vi "Actor Core.vi"(8 "error in":errorcluster, 11 "Select Report File Dialog in":refnum<class "Display Settings Dialog.lvclass">) -> (0 "error out":errorcluster, 3 "Actor out":refnum<class "Actor.lvclass">)   [LabVIEW 2014, in "Display Settings Dialog.lvlib" / "Display Settings Dialog.lvclass"]
doc: "(<B>Filename</B>: Actor Framework.lvlib:Actor.lvclass:Actor Core.vi)\n\nReceives messages to the actor, reacts to them, and initiates any error handling that may shut the actor down.\n\nDescendant classes may override this VI to append parallel tasks for the actor to complete while it handles messages. Overrides use the Call Parent Method node."
uses:
  Display Settings Dialog.lvclass
  <vilib>/ActorFramework/Actor/Actor.lvclass
  HIJ Vision Display/HIJ Vision Display/DisplaySettings.ctl
  <vilib>/ActorFramework/Actor/Actor.lvclass/Actor.ctl
  <vilib>/ActorFramework/Message Enqueuer/Message Enqueuer.lvclass/Message Enqueuer.ctl
  Display Settings Dialog.lvclass/Display Settings Dialog.ctl
  Display Settings Dialog Messages/Write Display settings Msg/Write Display settings Msg.lvclass/Write Display settings Msg.ctl
  HIJ Vision Display/HIJ Vision Display Messages/New Dispay Settings Msg/New Dispay Settings Msg.lvclass/New Dispay Settings Msg.ctl
  <vilib>/ActorFramework/Message Enqueuer/Init from Existing Queue.vi
  <vilib>/ActorFramework/Message Enqueuer/Enqueue.vi
  <vilib>/ActorFramework/Message Priority Queue/Priority Enqueue.vi
  <vilib>/ActorFramework/Message Enqueuer/Message Enqueuer.lvclass
  Display Settings Dialog Messages/Write Display settings Msg/Write Display settings Msg.lvclass
  HIJ Vision Display/HIJ Vision Display Messages/New Dispay Settings Msg/New Dispay Settings Msg.lvclass
  <vilib>/ActorFramework/Stop Msg/Stop Msg.lvclass
  Shared Code/Viewable Actor/ViewableActor/ViewableActor.lvclass
  HIJ Vision Display/HIJ Vision Display/HIJ Vision Display.lvclass
panel:
  in  "Display settings":T1={"Min. Thresh."=0.0, "X"=0.0, "Y"=0.0, "ShowLineout"=FALSE, "ScaleParts"=10, "ShowLegende"=FALSE, "Target Cross"=FALSE, "Centroid Cross"=FALSE, "Target color"=16777226, "Centroid color"=16711680, "calibr. µm/px"=0.0}
  in  "Stop Signal":bool
  in  "Stop":bool
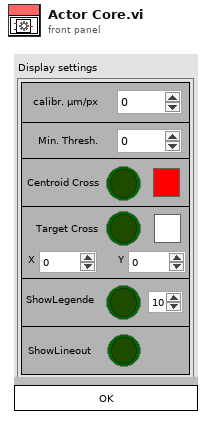
[diagram p1: front panel]
types:
  T1 = typedef "HIJ Vision Display.lvlib/HIJ Vision Display.lvclass/DisplaySettings.ctl" = cluster{"Min. Thresh.":sgl, "X":dbl, "Y":dbl, "ShowLineout":bool, "ScaleParts":i32, "ShowLegende":bool, "Target Cross":bool, "Centroid Cross":bool, "Target color":u32, "Centroid color":u32, "calibr. µm/px":sgl[unit]}
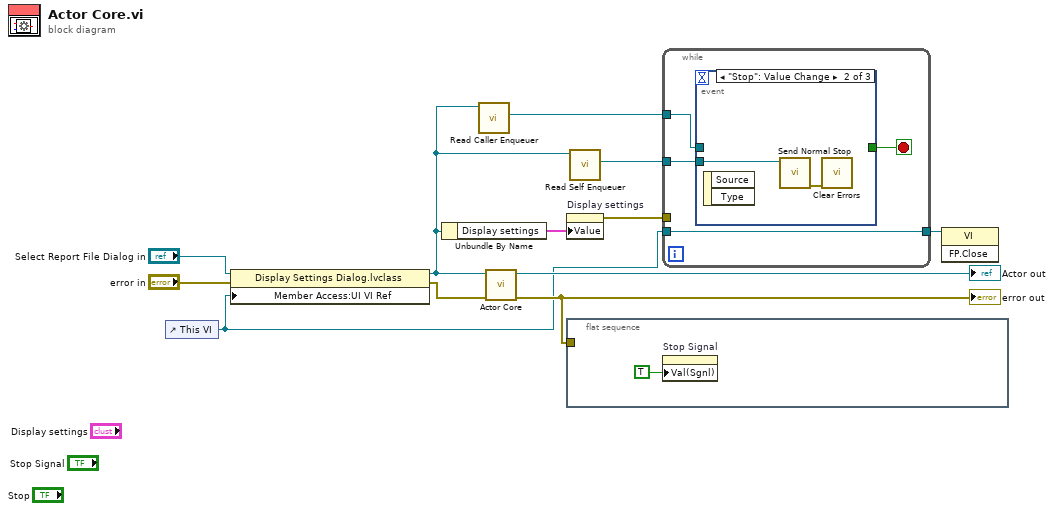
[diagram p0: block diagram]
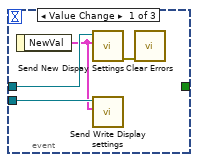
[diagram p2: hidden frame]
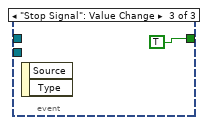
[diagram p3: hidden frame]
diagram:
  n1 = control-ref of="This VI"() -> (w3:refnum<vi>)
  n2 = property class="Display Settings Dialog.lvclass"(reference="Select Report File Dialog in", error in="error in", "Member Access:UI VI Ref"=w3) -> (reference out=w4:refnum<class "Display Settings Dialog.lvclass">, error out=w1:errorcluster)
  n3 = Unbundle By Name(w4) -> ("Display settings"=w6:T1)
  n4 = call <vilib>:"Read Caller Enqueuer.vi"("Actor"=w4) -> ("Caller Enqueuer"=w8:refnum<class "Message Enqueuer.lvclass">)  [unwired: 10 in]
  n5 = call-parent "Actor Core.vi"("error in"=w1, "Actor in"=w4) -> ("error out"=w11:errorcluster, "Actor out"=→"Actor out":refnum<class "Actor.lvclass">)  [unwired: 8 in]
  "error out" <- w11
  n6 = property on="Display settings" class="Clust (strict)"("Value"=w6) -> (error out=w5:errorcluster)  [unwired: 2 in, 1 out]
  n7 = flat-sequence {
    tunnel: w11 -> [_]
    frame #0 {
      n8 = property on="Stop Signal" class="Bool (strict)"("Val(Sgnl)"=TRUE ("Value (Signaling)")) -> ()  [unwired: 2 in, 2 out]
    }
  }
  n9 = call <vilib>:"Read Self Enqueuer.vi"("Actor"=w4) -> ("Self Enqueuer"=w10:refnum<class "Message Enqueuer.lvclass">)  [unwired: 10 in]
  n10 = while {
    tunnel: w10 -> [w17]
    tunnel: w3 -> [w15]
    tunnel: [w15] -> w9
    tunnel: w8 -> [w14]
    tunnel: w5 -> [_]
    stop <- w16 stop-if-true
    n11 = event shown="[1] \"Stop\": Value Change" {
      selector: _ -> [_ _ _]
      dyn-events: _ -> [_ _ _]
      timeout: _ -> [_ _ _]
      tunnel: w17 -> [w21 w23 _]
      tunnel: [_ _ TRUE] -> w16
      tunnel: w14 -> [w20 _ _]
      event Value Change {
        n12 = event-data() -> ("NewVal"=w19:T1)  [unwired: 1 in]
        n13 = call "Send New Dispay Settings.vi"("Display settings"=w19, "Message Enqueuer"=w20) -> ("error out"=w18:errorcluster)  [unwired: 8 in, 1 out]
        n14 = call "Send Write Display settings.vi"("Display settings"=w19, "Message Enqueuer"=w21) -> ()  [unwired: 8 in, 2 out]
        n15 = call <vilib>:"Clear Errors.vi"("error in (no error)"=w18) -> ()  [unwired: 5 in, 2 out]
      }
      event "Stop": Value Change {
        n16 = event-data() -> ()  [unwired: 1 in, 2 out]
        n17 = call <vilib>:"Send Normal Stop.vi"("Message Enqueuer"=w23) -> ("error out"=w22:errorcluster)  [unwired: 10 in]
        n18 = call <vilib>:"Clear Errors.vi"("error in (no error)"=w22) -> ()  [unwired: 5 in, 2 out]
      }
      event "Stop Signal": Value Change {
        n19 = event-data() -> ()  [unwired: 1 in, 2 out]
      }
    }
  }
  n20 = invoke class="VI" method="FP.Close"(reference=w9) -> ()  [unwired: 2 in, 3 out]
